vi "SelectionConfig.vi"(11 "GuiRef":T1={"StringOut"=refnum, "AbortOnFail"=refnum, "SN"=refnum, "SN_Length"=refnum, "TestResult"=refnum, "CycleTime"=refnum, "ErrorCode"=refnum, "UUTStatus"=refnum, "DataBaseEnable?"=refnum, "DUTModel"=refnum, "FixtureID"=refnum, "OperatorID"=refnum, "SNReady"=refnum, "StopSlot"=refnum, "NextStep"=refnum, "PassYeild"=refnum, "Failed"=refnum, "Passed"=refnum, "Tested"=refnum, "TestItemsCtl"={"StepName"="", "TestEnable"=FALSE, "LoopCount"=0, "StopOnFail"=FALSE, "Index"=0, "TestName"="", "通道"="", "参数"="", "TimeStart"=0}, "ProcessBar"=refnum, "Slot"=enum."Slot1", "Row"=3, "States"=refnum, "TestMode"=refnum, "循环次数-DUT"=refnum, "波形图"=refnum, "产品型号"=refnum, "子面板"=refnum, "测试失败项目"=refnum, "测试结果"=refnum, "DUT"=refnum, "Starttime"=refnum, "SlotReady"=refnum, "版本信息"=refnum}) -> (3 "CancelOut":bool)   [LabVIEW 2013]
uses:
  SysControl/Reference.ctl
  SysControl/TestItemsCTL.ctl
  SysControl/Slot.ctl
  SourceCode/GlobalValue.vi
  <vilib>/Utility/file.llb/Read From Spreadsheet File (string).vi
  <vilib>/Utility/file.llb/Write To Spreadsheet File (string).vi
panel:
  in  "SelectAll":bool
  in  "TestItems":i32(listbox)=1
  in  "Cancel":bool
  in  "Save":bool
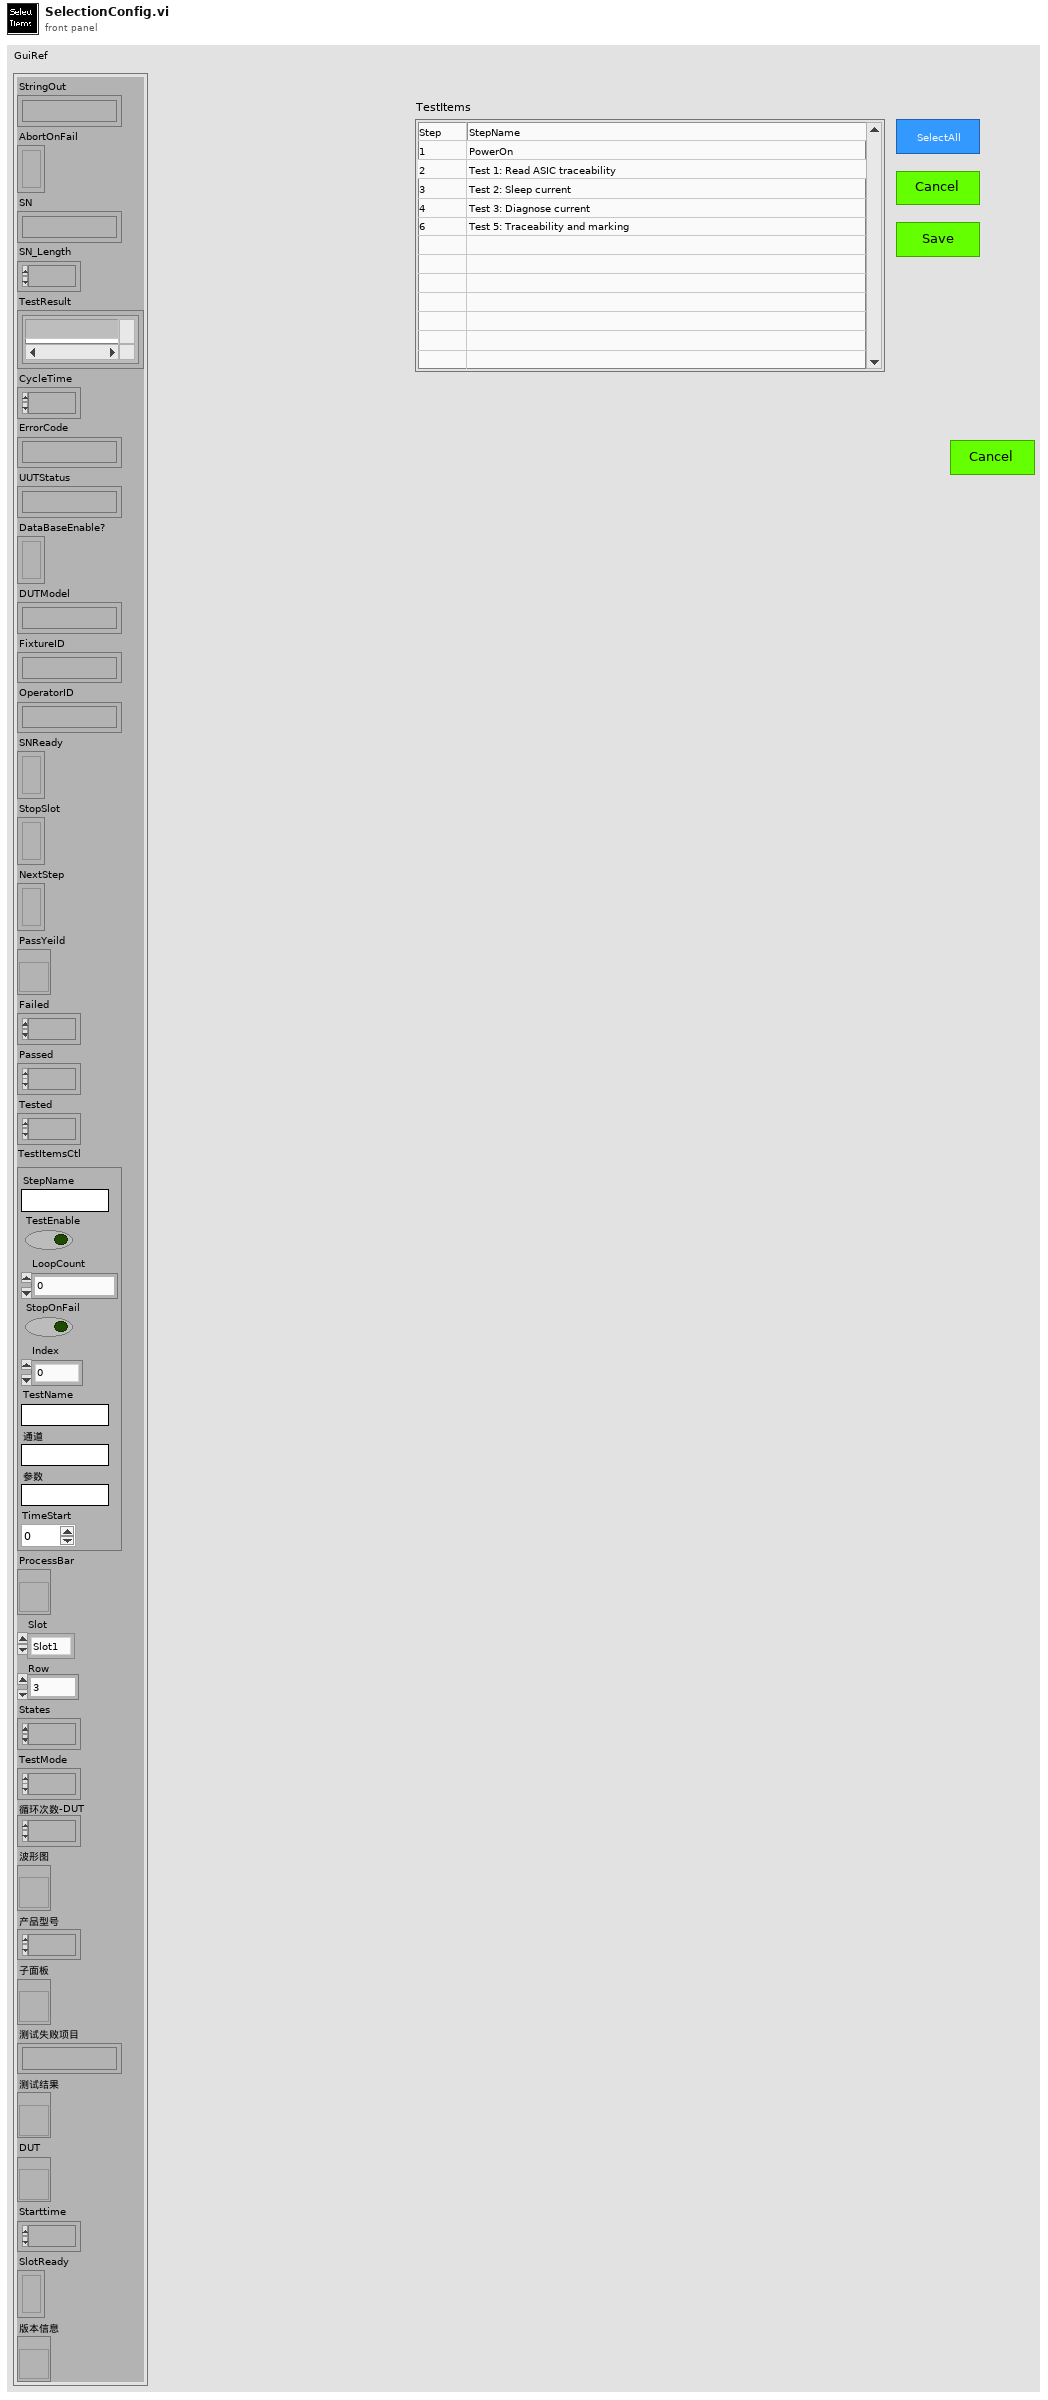
[diagram p1: front panel]
types:
  T1 = typedef "Reference.ctl" = cluster{"StringOut":refnum<vi>, "AbortOnFail":refnum<vi>, "SN":refnum<vi>, "SN_Length":refnum<vi>, "TestResult":refnum<vi>, "CycleTime":refnum<vi>, "ErrorCode":refnum<vi>, "UUTStatus":refnum<vi>, "DataBaseEnable?":refnum<vi>, "DUTModel":refnum<vi>, "FixtureID":refnum<vi>, "OperatorID":refnum<vi>, "SNReady":refnum<vi>, "StopSlot":refnum<vi>, "NextStep":refnum<vi>, "PassYeild":refnum<vi>, "Failed":refnum<vi>, "Passed":refnum<vi>, "Tested":refnum<vi>, "TestItemsCtl":T2, "ProcessBar":refnum<vi>, "Slot":T3, "Row":u32, "States":refnum<vi>, "TestMode":refnum<vi>, "循环次数-DUT":refnum<vi>, "波形图":refnum<vi>, "产品型号":refnum<vi>, "子面板":refnum<vi>, "测试失败项目":refnum<vi>, "测试结果":refnum<vi>, "DUT":refnum<vi>, "Starttime":refnum<vi>, "SlotReady":refnum<vi>, "版本信息":refnum<vi>}
  T2 = typedef "TestItemsCTL.ctl" = cluster{"StepName":string, "TestEnable":bool, "LoopCount":i32, "StopOnFail":bool, "Index":u32, "TestName":string, "通道":string, "参数":string, "TimeStart":u32}
  T3 = typedef "Slot.ctl" = enum16{"Slot1", "Slot2", "Slot3", "Slot4"}
  T4 = typedef "LVPoint32TypeDef.ctl" = cluster{"Horizontal":i32, "Vertical":i32}
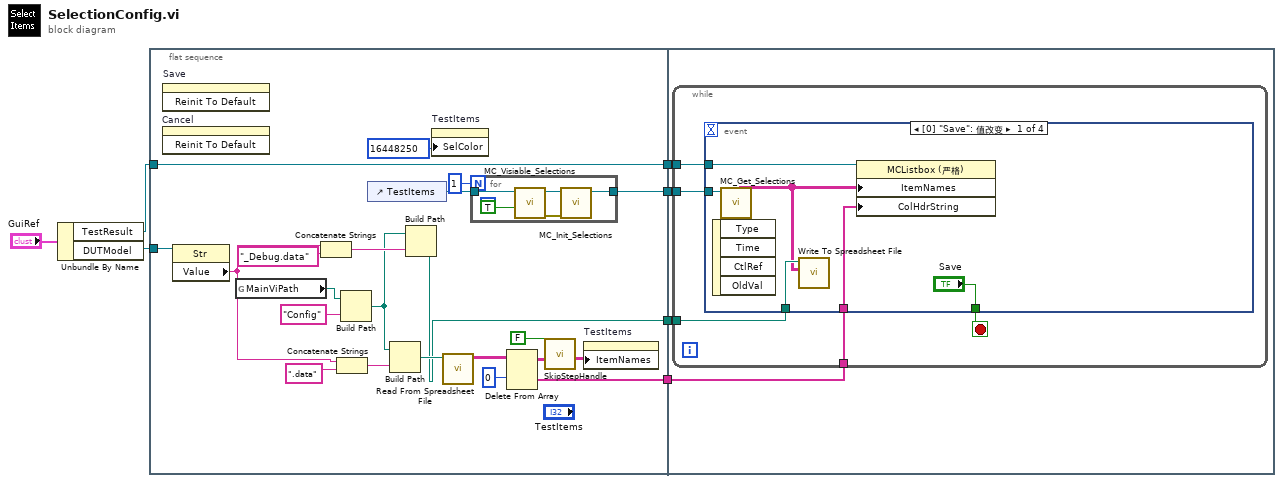
[diagram p0: block diagram]
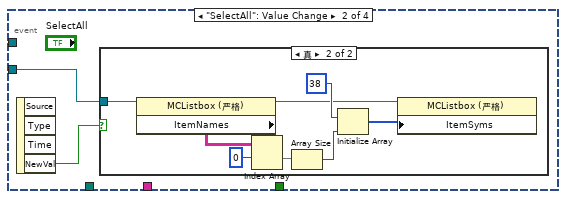
[diagram p2: hidden frame]
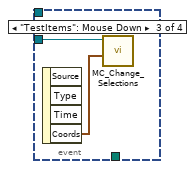
[diagram p4: hidden frame]
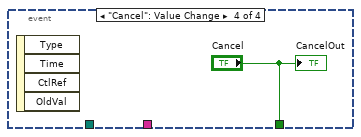
[diagram p5: hidden frame]
diagram:
  n1 = Unbundle By Name("GuiRef") -> ("TestResult"=w1:refnum<vi>, "DUTModel"=w3:refnum<vi>)
  n2 = flat-sequence {
    tunnel: [w18] -> w7
    tunnel: [w16] -> w6
    tunnel: [w12] -> w5
    tunnel: w3 -> [w11]
    tunnel: [w9] -> w2
    tunnel: w1 -> [w9]
    tunnel: w7 -> [w38]
    tunnel: w6 -> [w37]
    tunnel: w5 -> [w36]
    tunnel: w2 -> [w35]
    frame #0 {
      n3 = invoke on="Save" class="Bool" method="Reinit To Default"() -> ()  [unwired: 3 in, 3 out]
      n4 = invoke on="Cancel" class="Bool" method="Reinit To Default"() -> ()  [unwired: 3 in, 3 out]
      n5 = property class="Str"(reference=w11) -> ("Value"=w10:string)  [unwired: 1 in, 2 out]
      n6 = global read "GlobalValue.vi" "MainViPath"() -> (w8:path)
      n7 = Concatenate Strings(w10, "_Debug.data" ("名称或相对路径")) -> (w21:string)
      n8 = Concatenate Strings(w10, ".data" ("pattern (all files)")) -> (w27:string)
      n9 = Build Path(base path=w8, name or relative path="Config" ("名称或相对路径")) -> (appended path=w19:path)
      n10 = control-ref of="TestItems"() -> (w23:refnum<vi>)
      n11 = Build Path(base path=w19, name or relative path=w27) -> (appended path=w24:path)
      n12 = Build Path(base path=w19, name or relative path=w21) -> (appended path=w18:path)
      n13 = property on="TestItems" class="MCListbox (严格)"("SelColor"=u32 16448250 ("Selection Color")) -> ()  [unwired: 2 in, 2 out]
      n14 = call-poly <vilib>:"Read From Spreadsheet File.vi"("file path (dialog if empty)"=w24) -> ("all rows"=w25:string[][])  [unwired: 3 in, 7 out]
      n15 = for "For循环" {
        N: 1 -> [_]
        tunnel: w23 -> [w34]
        tunnel: [w30] -> w16
        n16 = call "MC_Visiable_Selections.vi"("VisiableSymbols"=TRUE, "MCin"=w34) -> ("error out"=w32:errorcluster, "MCout"=w33:refnum<vi>)  [unwired: 1 in, 7 out]
        n17 = call "MC_Init_Selections.vi"("error in (no error)"=w32, "MCin"=w33) -> ("MCout"=w30:refnum<vi>)  [unwired: 9 out]
      }
      n18 = Delete From Array(array=w25, index (row)=0 ("索引 (行)")) -> (deleted portion=w12:string[], array with subset deleted=w15:string[][])  [unwired: 2 in]
      n19 = call "SkipStepHandle.vi"("ItemNamesIn"=w15, "ShowSkipStep?"=FALSE) -> ("ItemNamesOut"=w13:string[][])  [unwired: 9 out]
      n20 = property on="TestItems" class="MCListbox (严格)"("ItemNames"=w13) -> ()  [unwired: 2 in, 2 out]
    }
    frame #1 {
      n21 = while {
        tunnel: w38 -> [w42]
        tunnel: w37 -> [w41]
        tunnel: w36 -> [w40]
        tunnel: w35 -> [w39]
        stop <- w43 stop-if-true
        n22 = event shown="[0] \"Save\": 值改变" {
          selector: _ -> [_ _ _ _]
          dyn-events: _ -> [_ _ _ _]
          timeout: _ -> [_ _ _ _]
          tunnel: ["Save" _ _ "Cancel"] -> w43
          tunnel: w42 -> [w49 _ _ _]
          tunnel: w41 -> [w48 w51 w61 _]
          tunnel: w40 -> [w47 _ _ _]
          tunnel: w39 -> [w44 _ _ _]
          event "Save": Value Change {
            n23 = event-data() -> ()  [unwired: 5 out]
            n24 = call "MC_Get_Selections.vi"("MCin"=w48) -> ("TestItems"=w46:string[][])  [unwired: 1 in, 9 out]
            n25 = call-poly <vilib>:"Write To Spreadsheet File.vi"("2D data"=w46, "file path (dialog if empty)"=w49) -> ()  [unwired: 4 in, 3 out]
            n26 = property on="属性节点" class="MCListbox (严格)"(reference=w44, "ItemNames"=w46, "ColHdrString"=w47) -> ()  [unwired: 1 in, 2 out]
          }
          event "SelectAll": Value Change {
            n27 = event-data() -> ("NewVal"=w50:bool)  [unwired: 4 out]
            n28 = case shown="真" w50 {
              tunnel: w51 -> [_ w54]
              frame False {
              }
              frame True {
                n29 = property on="属性节点" class="MCListbox (严格)"(reference=w54) -> (reference out=w52:refnum<vi>, "ItemNames"=w56:string[][])  [unwired: 1 in, 1 out]
                n30 = Index Array(array=w56, index (col)=0 ("index (row)")) -> (element=w57:string[])  [unwired: 1 in]
                n31 = Array Size(array=w57) -> (size(s)=w55:i32)
                n32 = Initialize Array(38, w55) -> (w58:i32[])
                n33 = property on="属性节点" class="MCListbox (严格)"(reference=w52, "ItemSyms"=w58) -> ()  [unwired: 1 in, 2 out]
              }
            }
          }
          event "TestItems": Mouse Down {
            n34 = event-data() -> ("Coords"=w60:T4)  [unwired: 4 out]
            n35 = call "MC_Change_Selections.vi"("Point"=w60, "MCin"=w61) -> ()  [unwired: 1 in, 9 out]
          }
          event "Cancel": Value Change {
            n36 = event-data() -> ()  [unwired: 5 out]
            "CancelOut" <- "Cancel"
          }
        }
      }
    }
  }
